vi "Close Session.vi"(0 "SLSC Remote in":refnum<class "SLSC Remote.lvclass">, 11 "error in (no error)":errorcluster) -> (15 "error out":errorcluster)   [LabVIEW 2016, in "SLSC Interfaces.lvlib" / "SLSC Remote.lvclass"]
uses:
  SLSC Remote.lvclass
  C:/Users/tblair/Documents/SLSC-Interface/Source/SLSC Interface Class/SLSC Interface.lvclass
  <vilib>/rajsite/i3-json/JSON Generation/Create Value Files/Create Value - Object.vi
  <vilib>/rajsite/i3-json/JSON Generation/Add Object Parameter Files/Add Object Parameter - String.vi
  <vilib>/NI/NI JSONRPC Server Framework/Classes/Server/Format Client Request (Auto-Increment).vi
  <vilib>/httpClient/POSTBuffer.vi
  <vilib>/NI/NI JSONRPC Server Framework/Classes/Server/JSONRPC Server.lvclass
  <vilib>/rajsite/i3-json/i3-json.lvlib
  <vilib>/httpClient/LabVIEWHTTPClient.lvlib
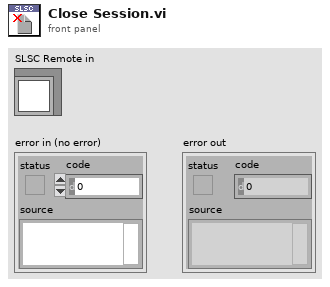
[diagram p1: front panel]
types:
  T1 = typedef "LabVIEWHTTPClient.lvlib/ClientHandle.ctl" = refnum<k1>
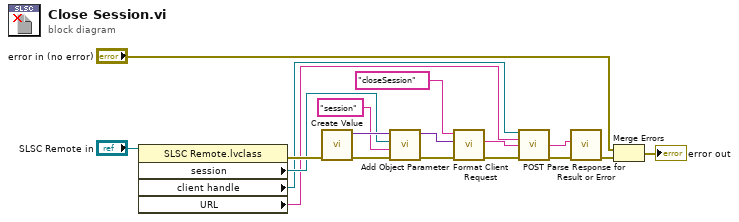
[diagram p0: block diagram]
diagram:
  n1 = property class="SLSC Remote.lvclass"(reference="SLSC Remote in") -> (error out=w16:errorcluster, "session"=w12:refnum<k21>, "client handle"=w8:T1, "URL"=w7:string)  [unwired: 1 in, 1 out]
  n2 = call-poly <vilib>:"Create Value.vi"("error in (no error)"=w16) -> ("error out"=w15:errorcluster, "JSON Tree"=w17:variant)  [unwired: 9 in]
  n3 = call-poly <vilib>:"Add Object Parameter.vi"("error in (no error)"=w15, "Name"="session", "String"=w12, "JSON Tree in (JSON Object)"=w17) -> ("error out"=w9:errorcluster, "JSON Tree out (JSON Object)"=w10:variant)  [unwired: 6 in]
  n4 = call-poly <vilib>:"Format Client Request.vi"("error in (no error)"=w9, "params"=w10, "method"="closeSession") -> ("error out"=w6:errorcluster, "Request String"=w13:string)  [unwired: 7 in]
  n5 = call-poly <vilib>:"POST.vi"("client handle"=w8, "url"=w7, "buffer"=w13, "error in (no error)"=w6) -> ("body"=w5:string, "error out"=w4:errorcluster)  [unwired: 8 in, 2 out]
  n6 = call <vilib>:"Parse Response for Result or Error.vi"("error in"=w4, "Response String In"=w5) -> ("error out"=w3:errorcluster)  [unwired: 7 in, 2 out]
  n7 = Merge Errors("error in (no error)", w3) -> (→"error out":errorcluster)
